vi "AddDatapoint.vi"(2 "error in (no error)":errorcluster, 3 "Location of DAQ":string, 4 "Temperature In":dbl, 5 "connection reference in":T1) -> (0 "error out":errorcluster, 1 "connection reference out":T1)   [LabVIEW 2023]
uses:
  <vilib>/addons/database/Connection.llb/Conn ObjectReference.ctl
  <vilib>/addons/database/Connection.llb/Conn Execute.vi
  <vilib>/addons/database/Recordset.llb/Rec Destroy - Connection.vi
  <vilib>/addons/database/NI_Database_API.lvlib
panel:
  # "In"
  # "Out"
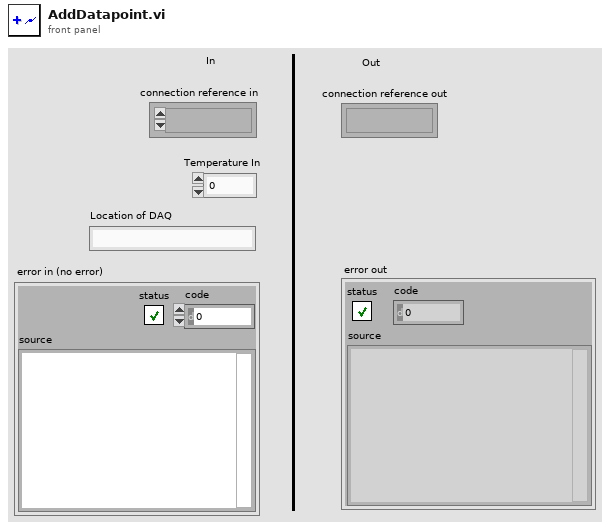
[diagram p1: front panel]
types:
  T1 = typedef "NI_Database_API.lvlib/Conn ObjectReference.ctl" = refnum<k1>
  T2 = typedef "NI_Database_API.lvlib/Rec ObjectReference.ctl" = refnum<k1>
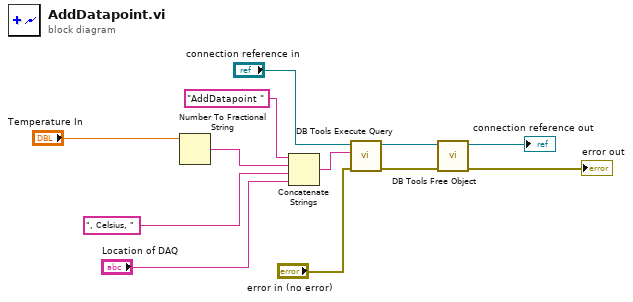
[diagram p0: block diagram]
diagram:
  n1 = Number To Fractional String(number="Temperature In") -> (F-format string=w10:string)  [unwired: 3 in]
  n2 = Concatenate Strings("AddDatapoint " ("string"), w10, ", Celsius, " ("string"), "Location of DAQ") -> (w9:string)
  n3 = call-poly <vilib>:"DB Tools Execute Query.vi"("error in (no error)"="error in (no error)", "SQL query"=w9, "connection reference"="connection reference in") -> ("error out"=w12:errorcluster, "recordset reference"=w11:T2)  [unwired: 5 in]
  n4 = call-poly <vilib>:"DB Tools Free Object.vi"("error in (no error)"=w12, "recordset reference"=w11) -> ("error out"=→"error out":errorcluster, "connection reference"=→"connection reference out":T1)  [unwired: 8 in]
